vi "Read Camera Enq.vi"(11 "HIJ Vision Camera App in":refnum<class "HIJ Vision Camera App.lvclass">) -> (2 "Actor Framework:Message Enqueuer":refnum<class "Message Enqueuer.lvclass">, 3 "HIJ Vision Camera App out":refnum<class "HIJ Vision Camera App.lvclass">)   [LabVIEW 2014, in "HIJ Vision Camera App.lvlib" / "HIJ Vision Camera App.lvclass"]
uses:
  HIJ Vision Camera App.lvclass
  <vilib>/ActorFramework/Message Enqueuer/Message Enqueuer.lvclass
  HIJ Vision Camera App.lvclass/HIJ Vision Camera App.ctl
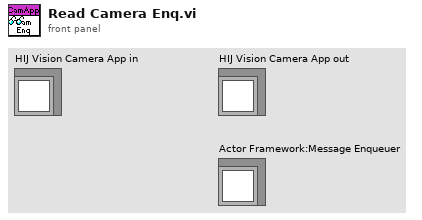
[diagram p1: front panel]
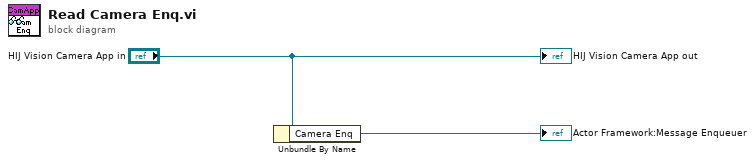
[diagram p0: block diagram]
diagram:
  n1 = Unbundle By Name("HIJ Vision Camera App in") -> ("Camera Enq"=→"Actor Framework:Message Enqueuer":refnum<class "Message Enqueuer.lvclass">)
  "HIJ Vision Camera App out" <- "HIJ Vision Camera App in"
